vi "Sub_Kalman_main.vi"(10 "Experiment":T1, 11 "KF":T2={"State"=[[1.0], [1.0]], "F state prop matrix"=[[1.0, 0.0], [0.0, 1.0]], "H measure matrix"=[[1.0, 0.0]], "P process cov"=[[1.0, 0.0], [0.0, 1.0]], "R measure cov"=[[1.0]], "Q state cov"=[], "T Sample"=0.1, "New Measurement"=10.0, "Measurement Variance"=0.2, "State Variance"=0.2, "Threshold"=0.4, "Initialized"=FALSE}) -> (2 "Experiment":T1, 3 "KF":T2={"State"=[[1.0], [0.0]], "F state prop matrix"=[[1.0, 0.0], [0.0, 1.0]], "H measure matrix"=[[1.0, 0.0]], "P process cov"=[], "R measure cov"=[], "Q state cov"=[], "T Sample"=0.0, "New Measurement"=0.0, "Measurement Variance"=0.0, "State Variance"=0.0, "Threshold"=0.0, "Initialized"=FALSE})   [LabVIEW 2021]
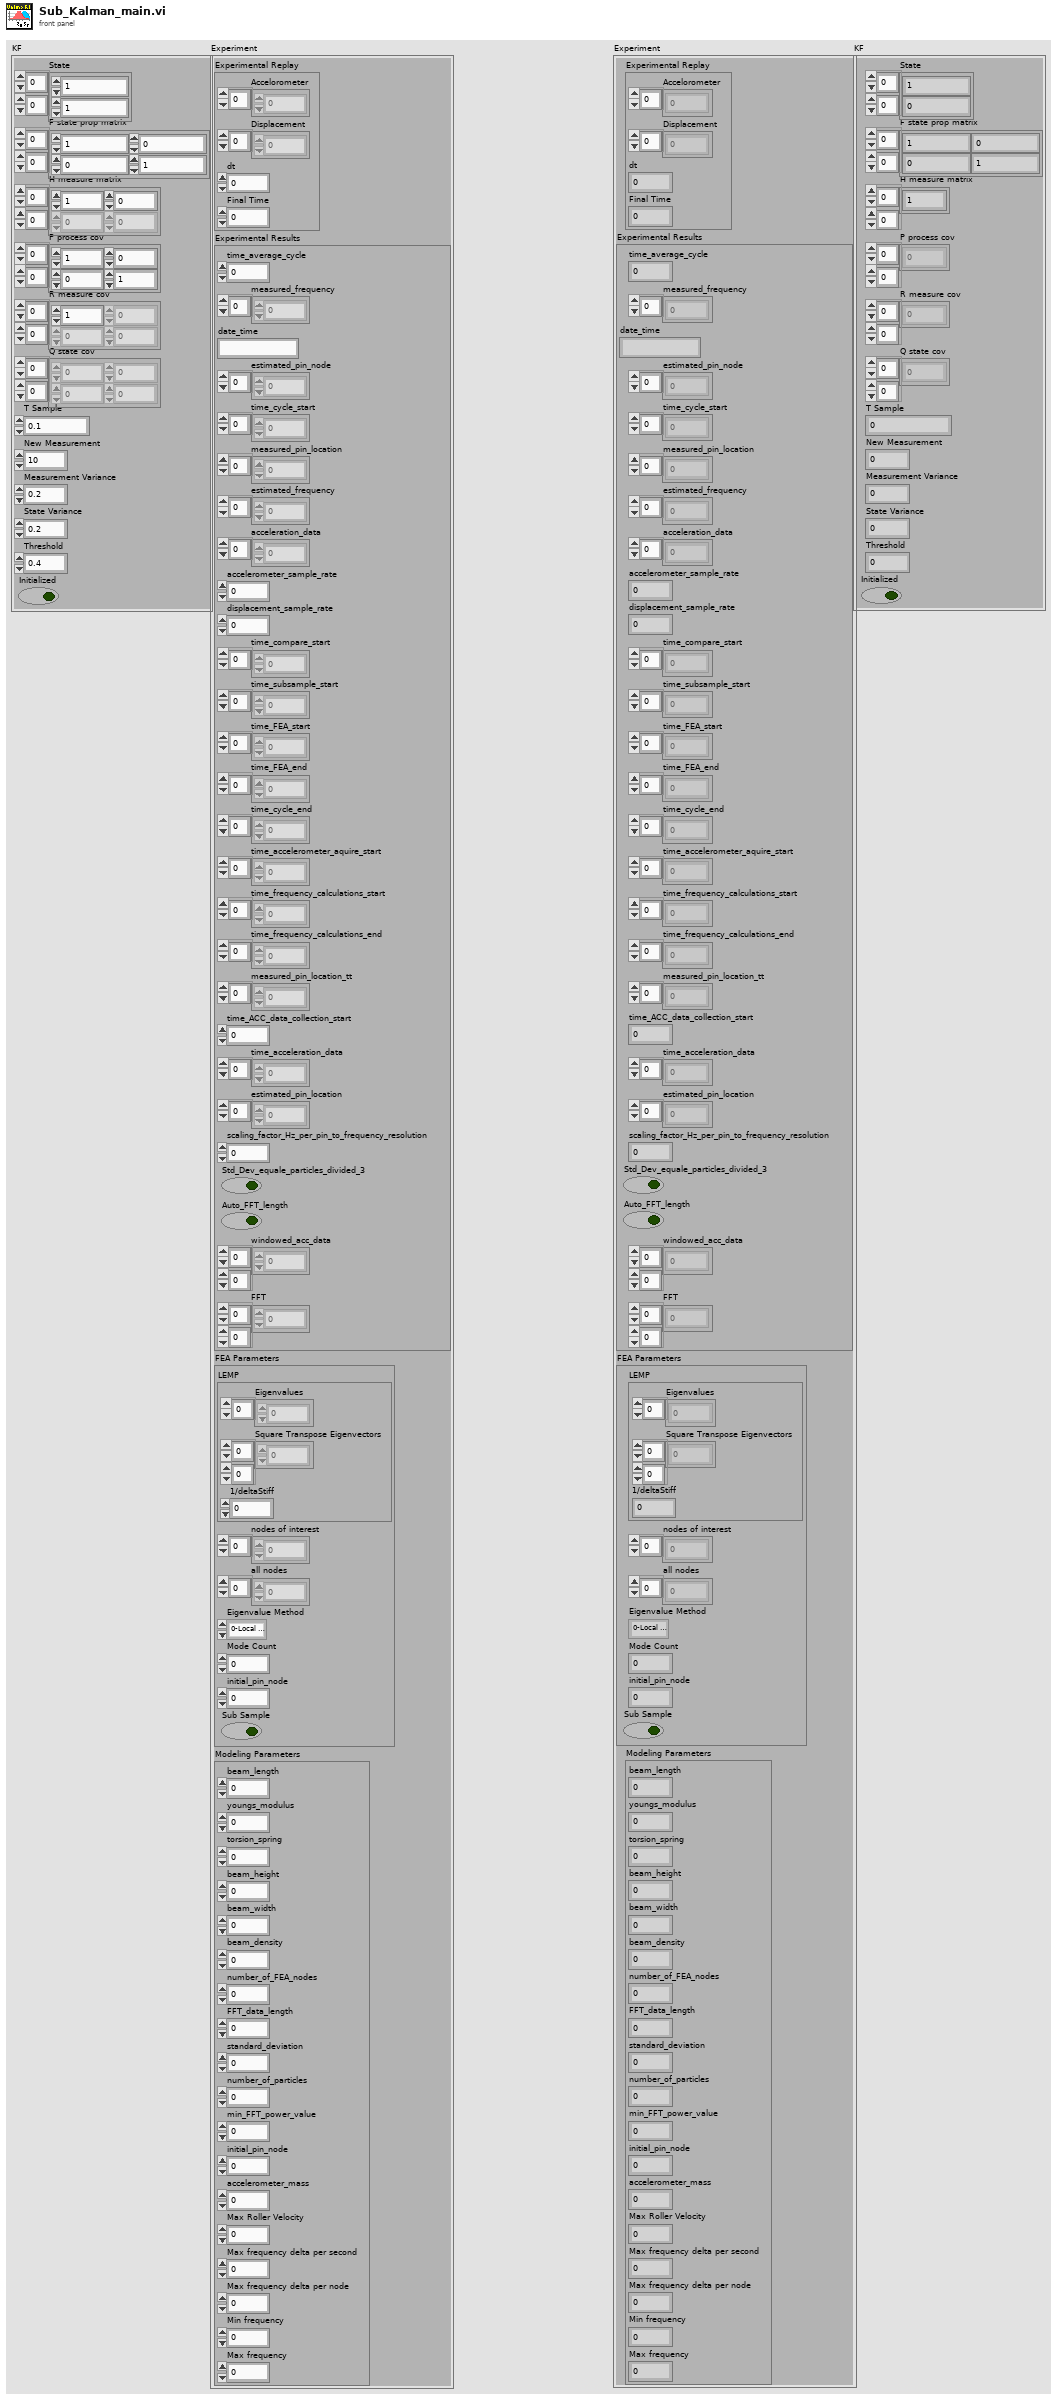
[diagram p1: front panel]
types:
  T1 = cluster{"Experimental Replay":cluster{"Accelorometer":dbl[], "Displacement":dbl[], "dt":dbl, "Final Time":dbl}, "Experimental Results":cluster{"time_average_cycle":dbl, "measured_frequency":dbl[], "date_time":string, "estimated_pin_node":i32[], "time_cycle_start":dbl[], "measured_pin_location":dbl[], "estimated_frequency":dbl[], "acceleration_data":dbl[], "accelerometer_sample_rate":dbl, "displacement_sample_rate":dbl, "time_compare_start":dbl[], "time_subsample_start":dbl[], "time_FEA_start":dbl[], "time_FEA_end":dbl[], "time_cycle_end":dbl[], "time_accelerometer_aquire_start":dbl[], "time_frequency_calculations_start":dbl[], "time_frequency_calculations_end":dbl[], "measured_pin_location_tt":dbl[], "time_ACC_data_collection_start":dbl, "time_acceleration_data":dbl[], "estimated_pin_location":dbl[], "scaling_factor_Hz_per_pin_to_frequency_resolution":dbl, "Std_Dev_equale_particles_divided_3":bool, "Auto_FFT_length":bool, "windowed_acc_data":dbl[][], "FFT":dbl[][]}, "FEA Parameters":cluster{"LEMP":cluster{"Eigenvalues":dbl[], "Square Transpose Eigenvectors":dbl[][], "1/deltaStiff":dbl}, "nodes of interest":i32[], "all nodes":i32[], "Eigenvalue Method":enum16{"0-Local Eigen Modification Procedure", "1-LabVIEW generalized eigenvalues", "2-LabVIEW M^-1K eigenvalues", "3-LabVIEW Cholesky Factorization", "4-Cholesky Factorization CPU SGL", "5-Cholesky Factorization CPU FXP", "6-Cholesky Factorization FPGA SGL", "7-Cholesky Factorization FPGA SGL SCL"}, "Mode Count":i32, "initial_pin_node":i32, "Sub Sample":bool}, "Modeling Parameters":cluster{"beam_length":dbl, "youngs_modulus":dbl, "torsion_spring":dbl, "beam_height":dbl, "beam_width":dbl, "beam_density":dbl, "number_of_FEA_nodes":i32, "FFT_data_length":i32, "standard_deviation":dbl, "number_of_particles":i32, "min_FFT_power_value":dbl, "initial_pin_node":i32, "accelerometer_mass":dbl, "Max Roller Velocity":dbl, "Max frequency delta per second":dbl, "Max frequency delta per node":dbl, "Min frequency":dbl, "Max frequency":dbl}}
  T2 = cluster{"State":dbl[][], "F state prop matrix":dbl[][], "H measure matrix":dbl[][], "P process cov":dbl[][], "R measure cov":dbl[][], "Q state cov":dbl[][], "T Sample":dbl, "New Measurement":dbl, "Measurement Variance":dbl, "State Variance":dbl, "Threshold":dbl, "Initialized":bool}
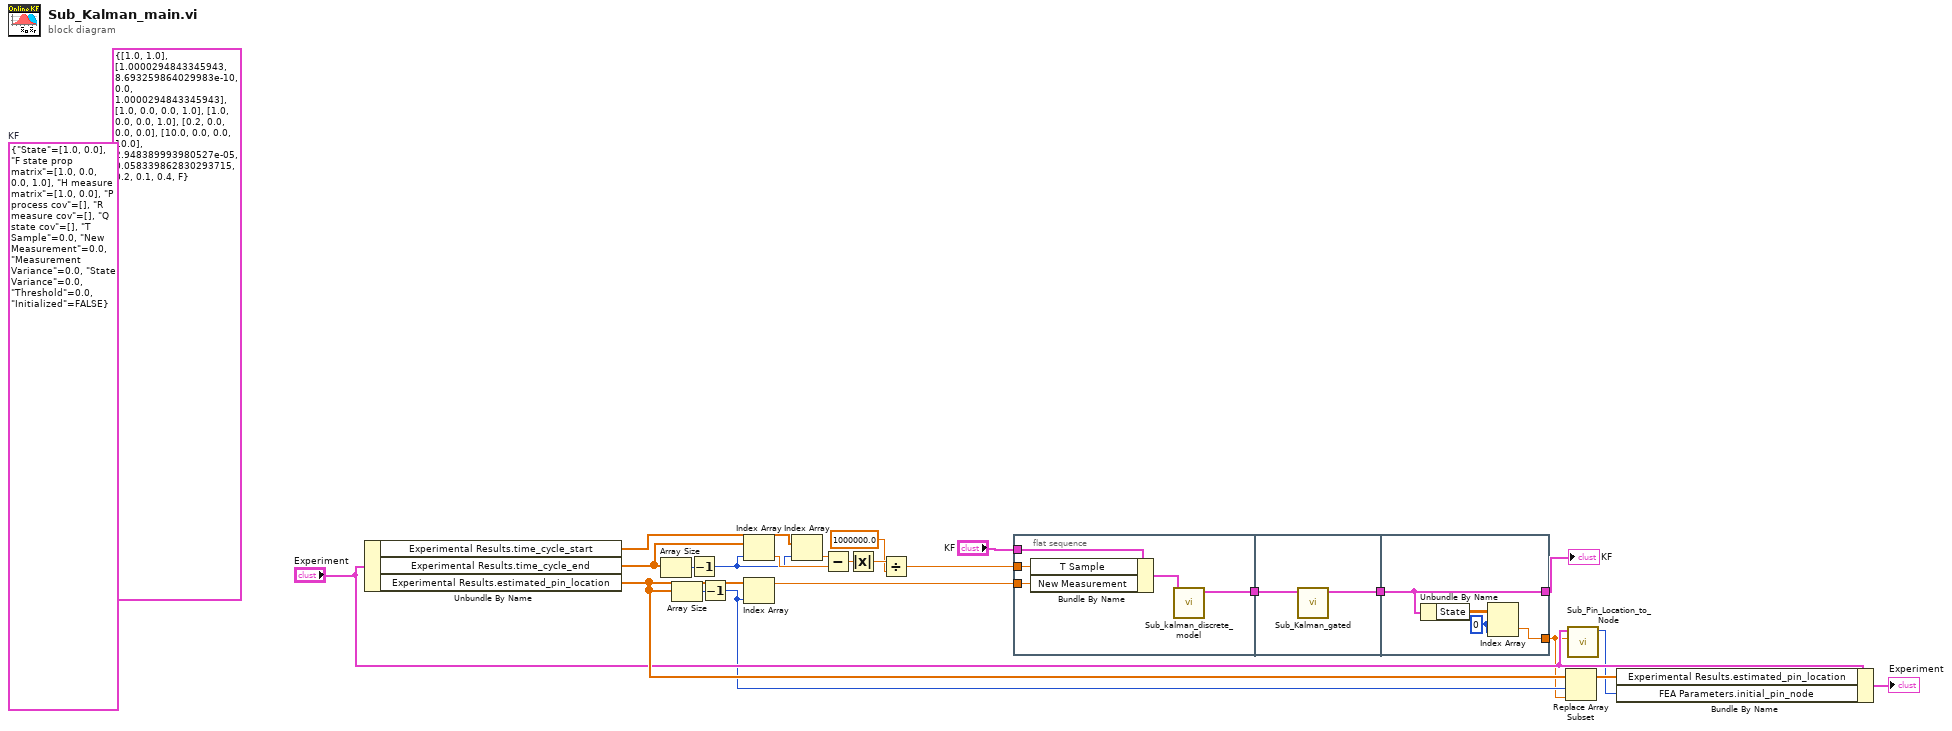
[diagram p0: block diagram]
diagram:
  (unwired) T2 {"State"=[[1.0], [1.0]], "F state prop matrix"=[[1.0000294843345943, 8.693259864029983e-10], [0.0, 1.0000294843345943]], "H measure matrix"=[[1.0, 0.0], [0.0, 1.0]], "P process cov"=[[1.0, 0.0], [0.0, 1.0]], "R measure cov"=[[0.2, 0.0], [0.0, 0.0]], "Q state cov"=[[10.0, 0.0], [0.0, 10.0]], "T Sample"=2.948389993980527e-05, "New Measurement"=0.058339862830293715, "Measurement Variance"=0.2, "State Variance"=0.1, "Threshold"=0.4, "Initialized"=FALSE} ("KF")
  (unwired) T2 {"State"=[[1.0], [0.0]], "F state prop matrix"=[[1.0, 0.0], [0.0, 1.0]], "H measure matrix"=[[1.0, 0.0]], "P process cov"=[], "R measure cov"=[], "Q state cov"=[], "T Sample"=0.0, "New Measurement"=0.0, "Measurement Variance"=0.0, "State Variance"=0.0, "Threshold"=0.0, "Initialized"=FALSE}  # KF
  n1 = Unbundle By Name("Experiment") -> ("Experimental Results.time_cycle_start"=w10:dbl[], "Experimental Results.time_cycle_end"=w3:dbl[], "Experimental Results.estimated_pin_location"=w19:dbl[])
  n2 = Array Size(array=w3) -> (size(s)=w4:i32)
  n3 = Array Size(array=w19) -> (size(s)=w20:i32)
  n4 = Decrement(x=w4) -> (x-1=w2:i32)
  n5 = Decrement(x=w20) -> (x-1=w6:i32)
  n6 = Index Array(array=w3, index=w2) -> (element=w13:dbl)
  n7 = Index Array(array=w19, index=w6) -> (element=w7:dbl)
  n8 = Index Array(array=w10, index=w2) -> (element=w14:dbl)
  n9 = Subtract(x=w14, y=w13) -> (x-y=w12:dbl)
  n10 = Absolute Value(x=w12) -> (abs(x)=w9:dbl)
  n11 = Divide(x=w9, y=1000000.0) -> (x/y=w1:dbl)
  n12 = flat-sequence {
    tunnel: [w27] -> w23
    tunnel: w1 -> [w26]
    tunnel: "KF" -> [w25]
    tunnel: w7 -> [w24]
    tunnel: w23 -> [w30]
    tunnel: [w29] -> w21
    tunnel: [w33] -> w22
    tunnel: w21 -> [w33]
    tunnel: [w31] -> w5
    frame #0 {
      n13 = Bundle By Name(cluster=w25, "T Sample"=w26, "New Measurement"=w24) -> (w28:T2)
      n14 = call "Sub_kalman_discrete_model.vi"("KF"=w28) -> ("KF"=w27:T2)  [unwired: 10 in]
    }
    frame #1 {
      n15 = call "Sub_Kalman_gated.vi"("KF"=w30) -> ("KF"=w29:T2)  [unwired: 10 in]
    }
    frame #2 {
      w32 = 0 ("index (row)")
      n16 = Unbundle By Name(w33) -> ("State"=w34:dbl[][])
      n17 = Index Array(array=w34, index (row)=w32, index (col)=w32) -> (element=w31:dbl)
    }
  }
  n18 = Replace Array Subset(array=w19, new element=w5, index=w6) -> (w18:dbl[])
  n19 = call "Sub_Pin_Location_to_Node.vi"("Pin Location"=w5, "Experiment in"="Experiment") -> ("DOF of Interest"=w15:i32)  [unwired: 9 in]
  n20 = Bundle By Name(cluster="Experiment", "Experimental Results.estimated_pin_location"=w18, "FEA Parameters.initial_pin_node"=w15) -> (→"Experiment":T1)
  "KF" <- w22
